vi "incrementActiveBridge.vi"(8 "error in (no error)":errorcluster, 11 "TestMonitor in":refnum<class "TestMonitor.lvclass">) -> (0 "error out":errorcluster, 3 "TestMonitor out":refnum<class "TestMonitor.lvclass">)   [LabVIEW 2013, in "TestMonitor.lvclass"]
uses:
  TestMonitor.lvclass
  TestMonitor.lvclass/TestMonitor.ctl
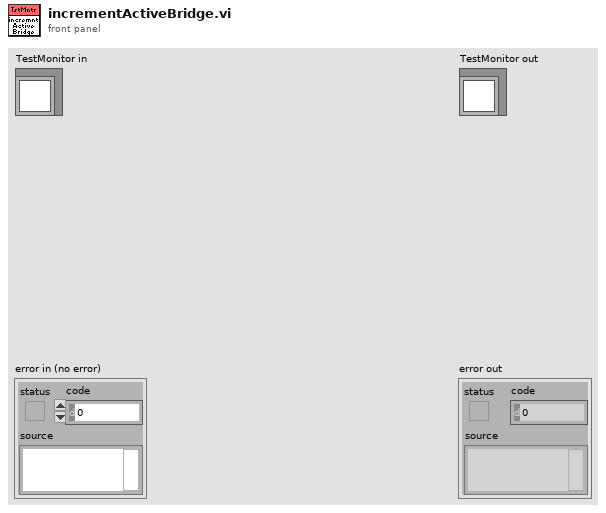
[diagram p1: front panel]
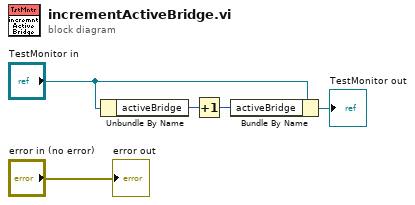
[diagram p0: block diagram]
diagram:
  n1 = Unbundle By Name("TestMonitor in") -> ("activeBridge"=w2:u32)
  n2 = Increment(x=w2) -> (x+1=w1:u32)
  n3 = Bundle By Name(cluster="TestMonitor in", "activeBridge"=w1) -> (→"TestMonitor out":refnum<class "TestMonitor.lvclass">)
  "error out" <- "error in (no error)"
